vi "arrays_examples.vi"() -> ()   [LabVIEW 2015]
doc: "Created by Artem Shevelev\nLabVIEW Portal profile: http://www.labviewportal.org/memberlist.php?mode=viewprofile&u=2340\ne-mail: artem.sh@gmail.com\nshevelev.pro"
uses:
  convertors/typedefs/BSONelement.ctl
  convertors/typedefs/dataType.ctl
  convertors/BSON_convertors_Library.lvlib
panel:
  out "value":variant
  out "data 2":T1[](array[typedef])
  out "arrayOfElements":T1[](array[typedef])
  out "BSONdoc":u8[](array[numeric]) format="%02x"
  out "error out":errorcluster
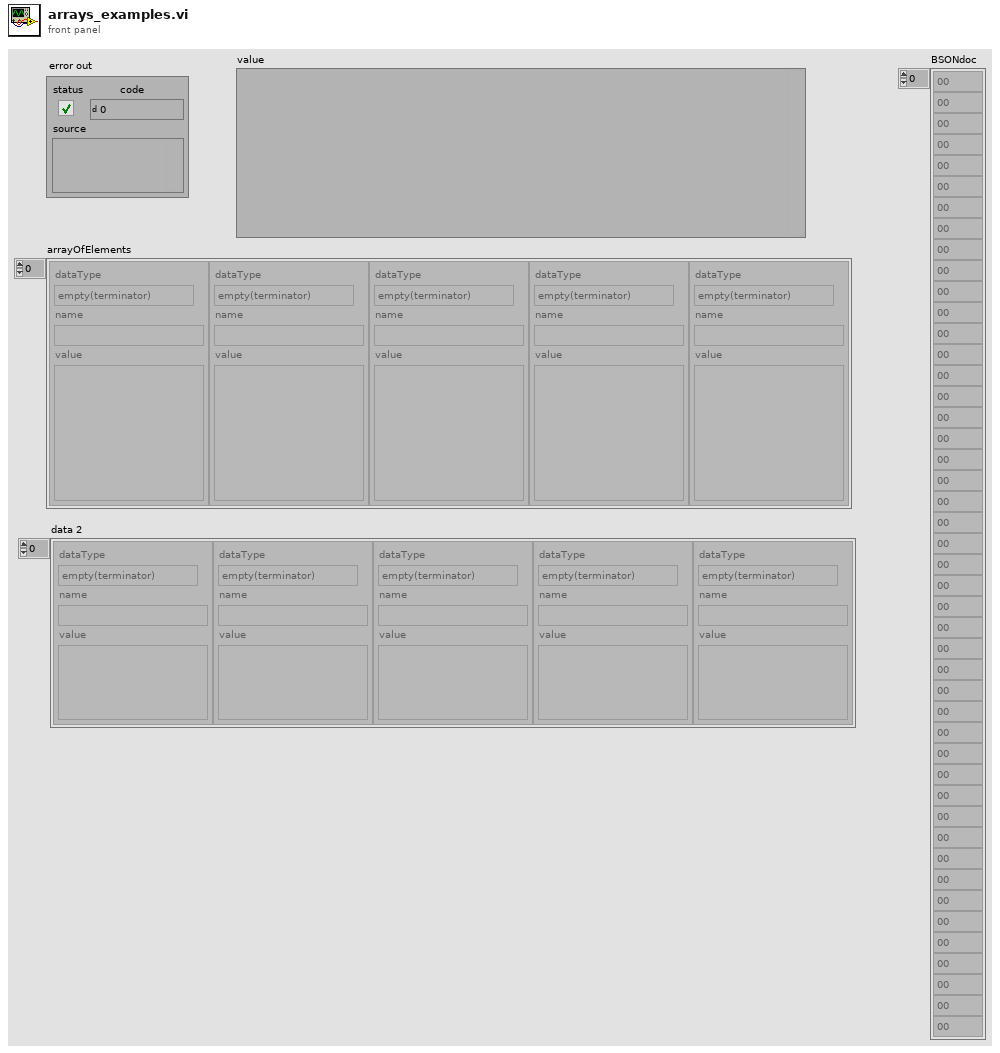
[diagram p1: front panel]
types:
  T1 = typedef "BSON_convertors_Library.lvlib/BSONelement.ctl" = cluster{"dataType":T2, "name":string, "value":variant}
  T2 = typedef "BSON_convertors_Library.lvlib/dataType.ctl" = enum8{"empty(terminator)", "double", "string", "document", "array", "binary", "Deprecated(Undefined)", "ObjectId", "boolean", "UTC datetime", "Null value", "cstring", "Deprecated(DBPointer)", "JavaScript", "Deprecated(Symbol)", "code_w_s", "int32", "uint64", "int64", "ext (decimal128)", "Min key", "Max key"}
  T3 = cluster{"lenngg":i32, "strArray":u64[], "clusterIn":cluster{"lenn1":i32, "lenn2":i32}, "lastStr":string, "lastStr 2":string}
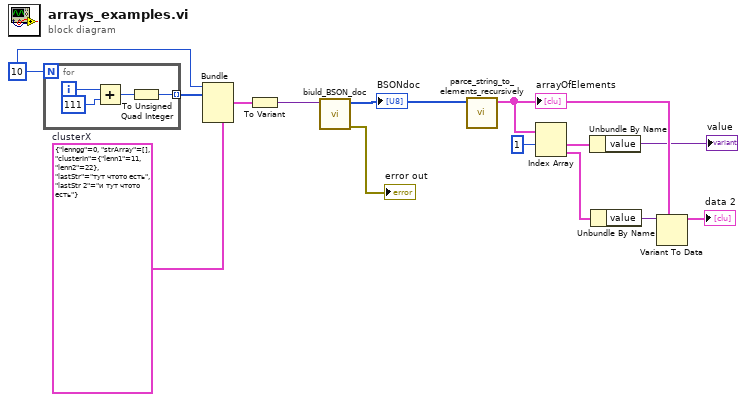
[diagram p0: block diagram]
diagram:
  w10 = T3 {"lenngg"=0, "strArray"=[], "clusterIn"={"lenn1"=11, "lenn2"=22}, "lastStr"="тут чтото есть", "lastStr 2"="и тут чтото есть"}  # clusterX
  w13 = 10
  n1 = for {
    N: w13 -> [_]
    tunnel: [w17] -> w3 mode=indexing
    i -> [w18]
    n2 = Add(x=w18, y=111) -> (x+y=w15:i32)
    n3 = To Unsigned Quad Integer(1:w15) -> (0:w17:u64)
  }
  n4 = Bundle(cluster=w10, "lenngg"=w13, "strArray"=w3) -> (w12:T3)  [unwired: 3 in]
  n5 = To Variant(anything=w12) -> (Variant=w11:variant)
  n6 = call "biuld_BSON_doc.vi"("data"=w11) -> ("error out"=→"error out":errorcluster, "BSONdoc"=w9:u8[])  [unwired: 9 in]
  "BSONdoc" <- w9
  n7 = call "parce_string_to_elements_recursively.vi"("BSONdoc"=w9) -> ("arrayOfElements"=w2:T1[])  [unwired: 9 in, 1 out]
  "arrayOfElements" <- w2
  n8 = Index Array(array=w2, index #1=1 ("index")) -> (element #1=w7:T1, element #2=w6:T1)  [unwired: 1 in]
  n9 = Unbundle By Name(w7) -> ("value"=→"value":variant)
  n10 = Unbundle By Name(w6) -> ("value"=w5:variant)
  n11 = Variant To Data(type=w2, Variant=w5) -> (data=→"data 2":T1[])  [unwired: 1 in, 1 out]
